vi "CreateObstacleOurRobots.vi"(0 "field_length":u32, 1 "grid in":T1, 2 "dy in":dbl[](array[numeric])=[1.0, -1.0, 0.0, 0.0, 1.0, -1.0, 1.0, -1.0], 5 "field_width":u32, 7 "dx in":dbl[](array[numeric])=[0.0, 0.0, 1.0, -1.0, 1.0, 1.0, -1.0, -1.0], 9 "n horizontal":dbl, 11 "ClosedSet in":dbl[][](array[numeric]), 12 "our robots":T2[](array[typedef]), 13 "n vertical":dbl, 14 "GridParameter":dbl) -> (6 "grid out":T1, 8 "ClosedSet out":dbl[][](array[numeric]))   [LabVIEW 2016]
uses:
  Core/AI Robot.ctl
  Intel/Functions Enum.ctl
  Intel/AttackerStates.ctl
  grid.ctl
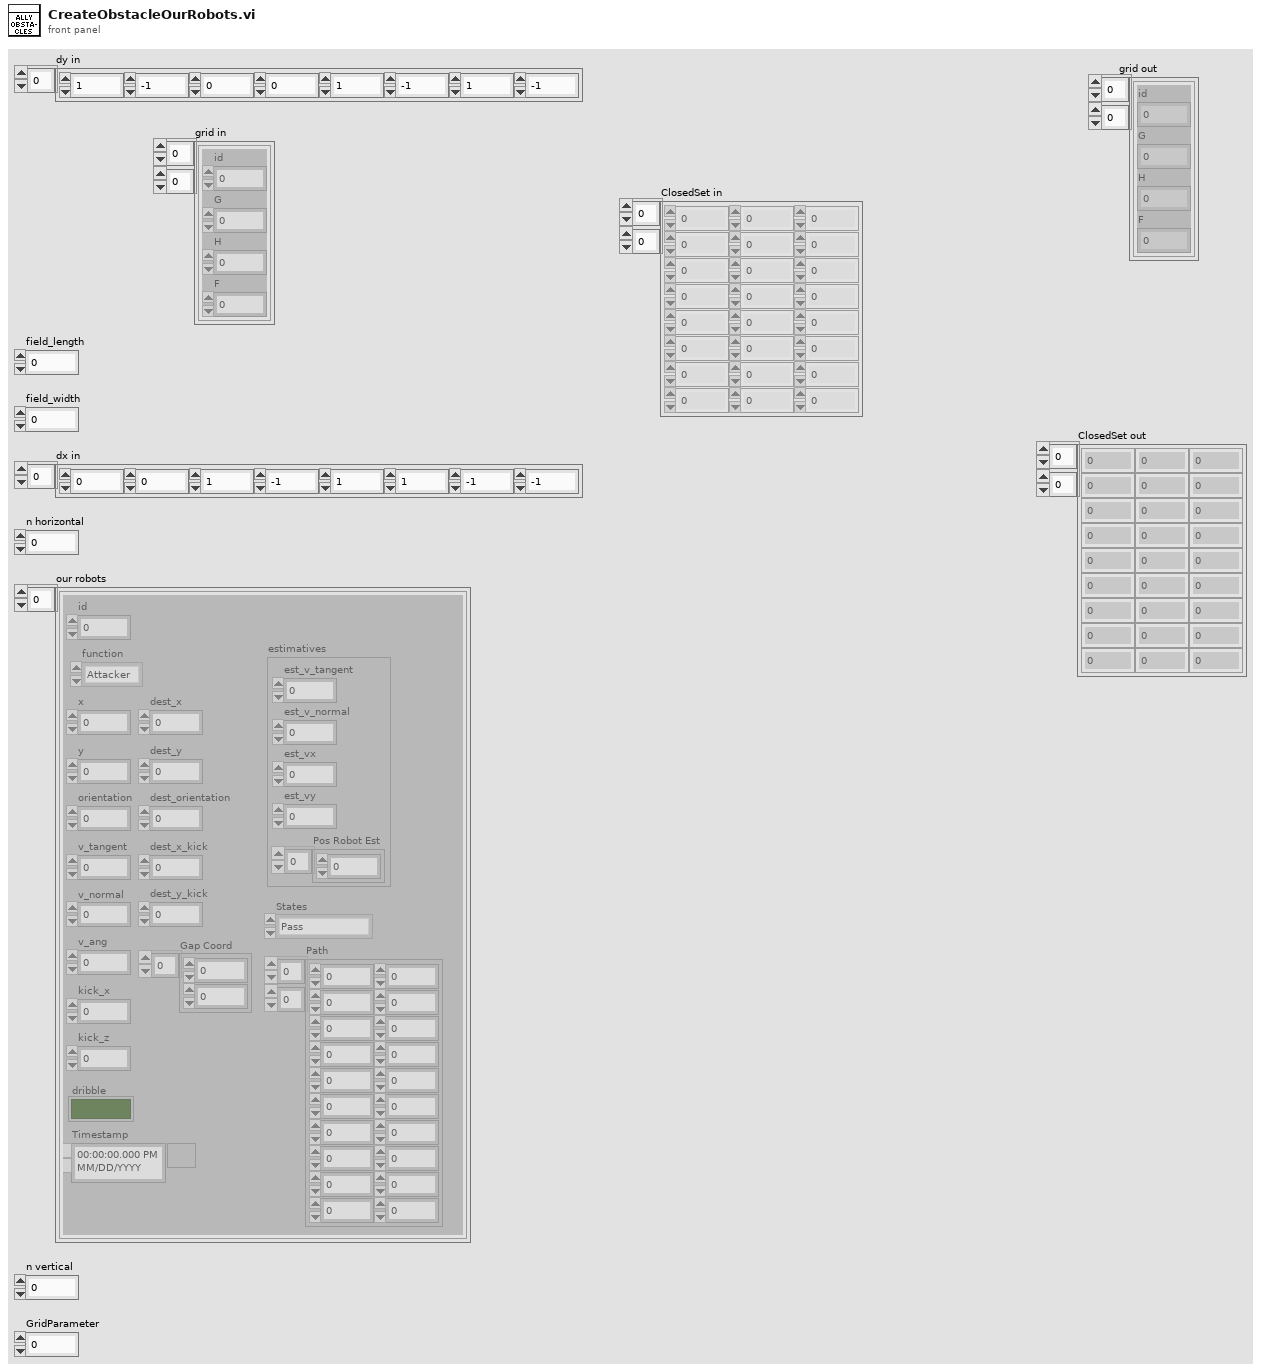
[diagram p1: front panel]
types:
  T1 = typedef "grid.ctl" = cluster{"id":dbl, "G":dbl, "H":dbl, "F":dbl}[][]
  T2 = typedef "AI Robot.ctl" = cluster{"id":u32, "function":T3, "x":dbl, "y":dbl, "orientation":dbl, "v_tangent":dbl, "v_normal":dbl, "v_ang":dbl, "kick_x":dbl, "kick_z":dbl, "dribble":bool, "Timestamp":timestamp, "dest_x":dbl, "dest_y":dbl, "dest_orientation":dbl, "estimatives":cluster{"est_v_tangent":dbl, "est_v_normal":dbl, "est_vx":dbl, "est_vy":dbl, "Pos Robot Est":dbl[]}, "dest_x_kick":dbl, "dest_y_kick":dbl, "Gap Coord":dbl[], "States":T4, "Path ":dbl[][]}
  T3 = typedef "Functions Enum.ctl" = enum16{"Attacker", "Goalie", "Defender", "Striker", "Goto 0", "Dummy", "Kicker", "ZigZag"}
  T4 = typedef "AttackerStates.ctl" = enum16{"Pass", "GoToTangent", "BallGetting", "GoToKick", ""}
  T5 = cluster{"[0]":dbl, "[1]":dbl, "[2]":dbl, "[3]":dbl}
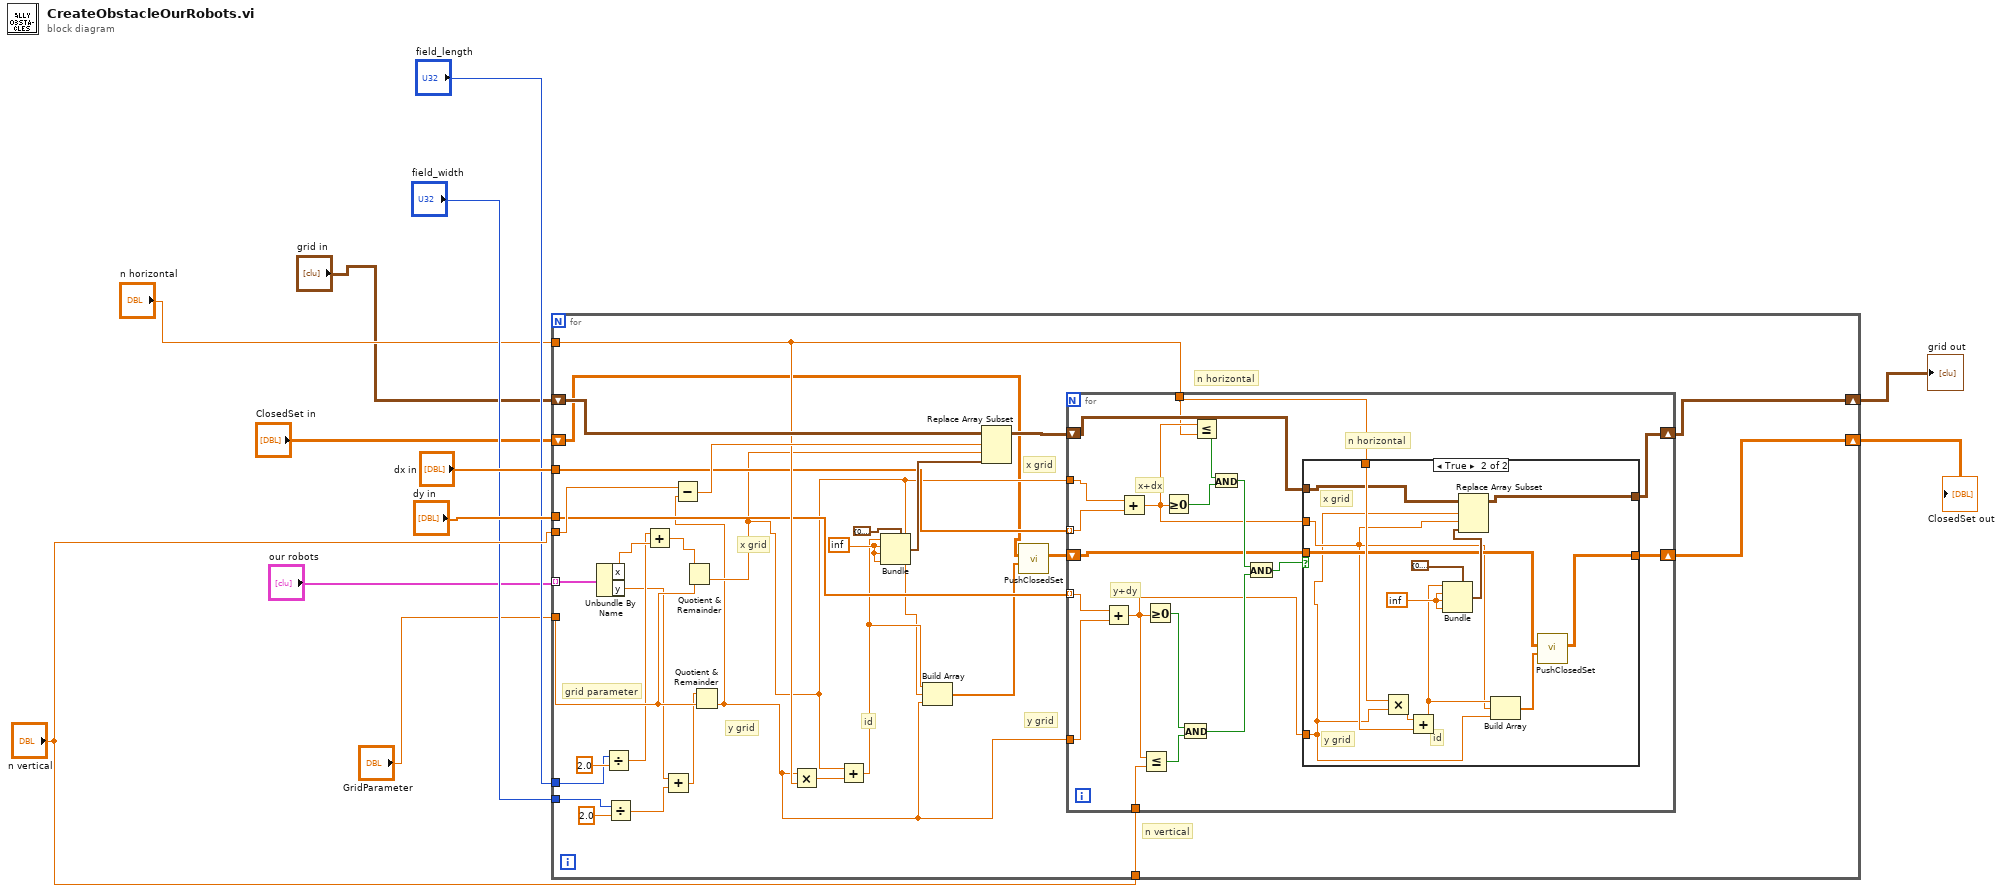
[diagram p0: block diagram]
diagram:
  n1 = for {
    shift-right: [w22] -> w1
    shift-left: "grid in" -> [w42]
    tunnel: "our robots" -> [w44] mode=indexing
    tunnel: "GridParameter" -> [w43]
    tunnel: "field_length" -> [w36]
    tunnel: "field_width" -> [w37]
    tunnel: "n vertical" -> [w31]
    tunnel: "n horizontal" -> [w24]
    tunnel: "n vertical" -> [w23]
    tunnel: "dx in" -> [w21]
    tunnel: "dy in" -> [w20]
    shift-right: [w13] -> w3
    shift-left: "ClosedSet in" -> [w14]
    w27 = inf
    # "n vertical"
    # "n horizontal"
    # "y grid"
    # "x grid"
    # "id"
    # "y grid"
    # "x grid"
    # "grid parameter"
    n2 = Unbundle By Name(w44) -> ("x"=w40:dbl, "y"=w33:dbl)
    n3 = Divide(x=w36, y=2.0) -> (x/y=w35:dbl)
    n4 = Divide(x=w37, y=2.0) -> (x/y=w34:dbl)
    n5 = Add(x=w35, y=w40) -> (x+y=w41:dbl)
    n6 = Add(x=w33, y=w34) -> (x+y=w32:dbl)
    n7 = Quotient & Remainder(x=w41, y=w43) -> (floor(x/y)=w18:dbl)  [unwired: 1 out]
    n8 = Quotient & Remainder(x=w32, y=w43) -> (floor(x/y)=w17:dbl)  [unwired: 1 out]
    n9 = Subtract(x=w31, y=w17) -> (x-y=w29:dbl)
    n10 = Multiply(x=w17, y=w24) -> (x*y=w28:dbl)
    n11 = Add(x=w18, y=w28) -> (x+y=w19:dbl)
    n12 = Bundle(cluster=T5 {"[0]"=0.0, "[1]"=0.0, "[2]"=0.0, "[3]"=0.0} ("element 2"), "[0]"=w19, "[1]"=w27, "[2]"=w27, "[3]"=w27) -> (w26:T5)
    n13 = Build Array(w19, w18, w17) -> (w16:dbl[])
    n14 = Replace Array Subset(array=w42, new element=w26, index (row)=w29, index (col)=w18) -> (w25:T1)
    n15 = call "PushClosedSet.vi"("Novo nó"=w16, "ClosedSet"=w14) -> ("NewClosedSet"=w15:dbl[][])  [unwired: 9 in]
    n16 = for {
      tunnel: w21 -> [w63] mode=indexing
      tunnel: w20 -> [w62] mode=indexing
      tunnel: w18 -> [w52]
      tunnel: w17 -> [w51]
      tunnel: w24 -> [w48]
      tunnel: w23 -> [w59]
      shift-right: [w47] -> w22
      shift-left: w25 -> [w53]
      shift-right: [w45] -> w13
      shift-left: w15 -> [w46]
      # "y+dy"
      # "x+dx"
      # "n horizontal"
      n17 = Add(x=w62, y=w51) -> (x+y=w49:dbl)
      n18 = Add(x=w52, y=w63) -> (x+y=w50:dbl)
      n19 = Less Or Equal?(x=w49, y=w59) -> (x <= y?=w57:bool)
      n20 = Greater Or Equal To 0?(x=w49) -> (x >= 0?=w58:bool)
      n21 = Greater Or Equal To 0?(x=w50) -> (x >= 0?=w60:bool)
      n22 = And(x=w58, y=w57) -> (x .and. y?=w55:bool)
      n23 = Less Or Equal?(x=w50, y=w48) -> (x <= y?=w61:bool)
      n24 = And(x=w61, y=w60) -> (x .and. y?=w56:bool)
      n25 = And(x=w56, y=w55) -> (x .and. y?=w54:bool)
      n26 = case shown="True" w54 {
        tunnel: w53 -> [w65 w73]
        tunnel: [w65 w72] -> w47
        tunnel: w50 -> [_ w68]
        tunnel: w49 -> [_ w67]
        tunnel: w48 -> [_ w75]
        tunnel: w46 -> [w64 w71]
        tunnel: [w64 w70] -> w45
        frame False {
        }
        frame True {
          w77 = inf
          # "id"
          # "x grid"
          # "y grid"
          n27 = Multiply(x=w75, y=w67) -> (x*y=w74:dbl)
          n28 = Add(x=w74, y=w68) -> (x+y=w69:dbl)
          n29 = Bundle(cluster=T5 {"[0]"=0.0, "[1]"=0.0, "[2]"=0.0, "[3]"=0.0} ("element 2"), "[0]"=w69, "[1]"=w77, "[2]"=w77, "[3]"=w77) -> (w76:T5)
          n30 = Replace Array Subset(array=w73, new element=w76, index (row)=w67, index (col)=w68) -> (w72:T1)
          n31 = Build Array(w69, w68, w67) -> (w66:dbl[])
          n32 = call "PushClosedSet.vi"("Novo nó"=w66, "ClosedSet"=w71) -> ("NewClosedSet"=w70:dbl[][])  [unwired: 9 in]
        }
      }
    }
  }
  "ClosedSet out" <- w3
  "grid out" <- w1
